vi "SumAbs.vi"(11 "Array In":dbl[][](array[numeric])) -> (3 "sum":dbl)   [LabVIEW 2018]
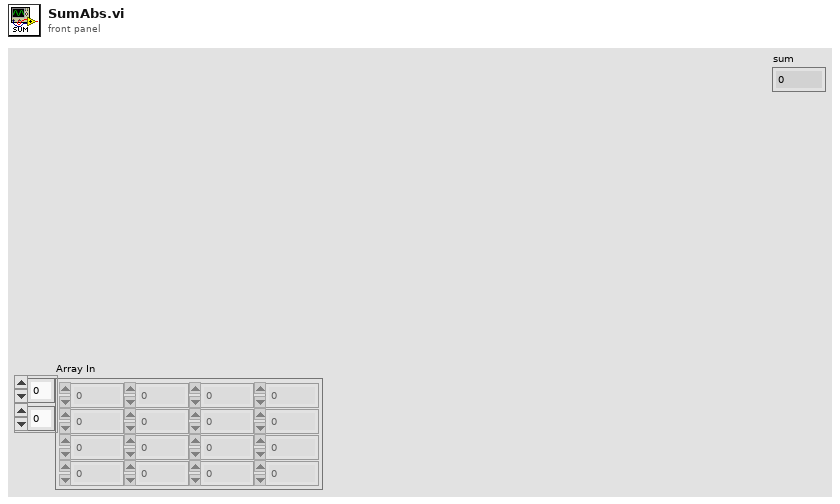
[diagram p1: front panel]
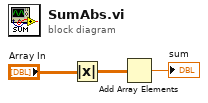
[diagram p0: block diagram]
diagram:
  n1 = Absolute Value(x="Array In") -> (abs(x)=w2:dbl[][])
  n2 = Add Array Elements(numeric array=w2) -> (sum=→"sum":dbl)
